vi "Read DDS Writer Object.vi"(11 "Device DDS Communications in":refnum<class "Device DDS Communications.lvclass">) -> (2 "DDS Writer Object":refnum<class "DDS Writer.lvclass">, 3 "Device DDS Communications out":refnum<class "Device DDS Communications.lvclass">)   [LabVIEW 2018, in "Device DDS Communications Framework.lvlib" / "Device DDS Communications.lvclass"]
uses:
  Device DDS Communications.lvclass
  <vilib>/ORNL/CSEISMIC DDS/DDS Writer/DDS Writer.lvclass
  Device DDS Communications.lvclass/Device DDS Communications.ctl
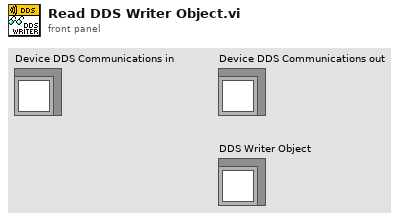
[diagram p1: front panel]
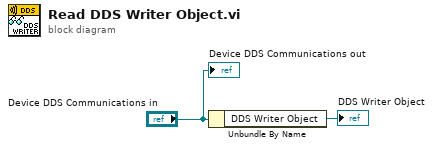
[diagram p0: block diagram]
diagram:
  n1 = Unbundle By Name("Device DDS Communications in") -> ("DDS Writer Object"=→"DDS Writer Object":refnum<class "DDS Writer.lvclass">)
  "Device DDS Communications out" <- "Device DDS Communications in"
